vi "LV2015_PC_Build SD Card LED File from Page Cluser Array.vi"(7 "file path (dialog if empty)":path, 9 "pixel Count":u32=70, 11 "LED File Array":T1[](array[typedef])) -> ()   [LabVIEW 2016]
uses:
  TypeDefs/Cluster_Page Data.ctl
  <vilib>/Utility/file.llb/Write Delimited Spreadsheet (I64).vi
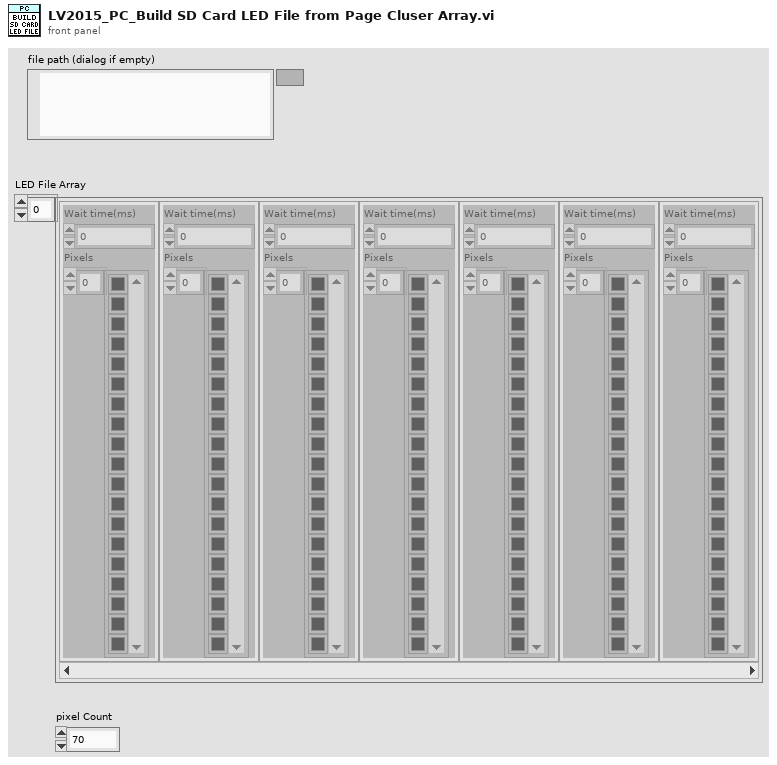
[diagram p1: front panel]
types:
  T1 = typedef "Cluster_Page Data.ctl" = cluster{"Wait time(ms)":u32, "Pixels":u32[]}
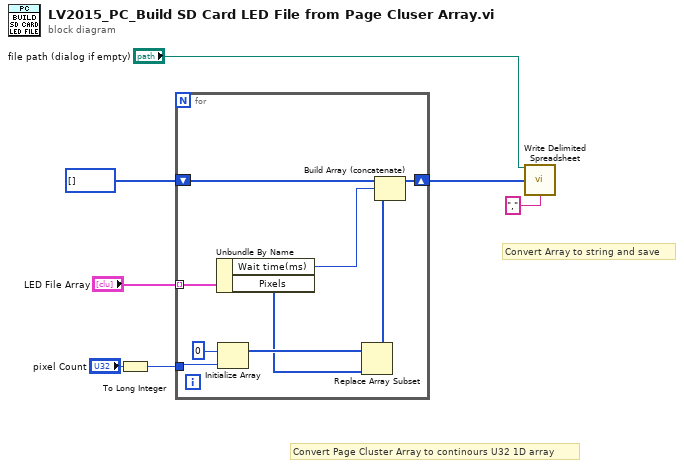
[diagram p0: block diagram]
diagram:
  # "Convert Array to string and save"
  # "Convert Page Cluster Array to continours U32 1D array"
  n1 = To Long Integer(number="pixel Count") -> (32bit integer=w4:i32)
  n2 = for {
    tunnel: "LED File Array" -> [w14] mode=indexing
    shift-right: [w10] -> w3
    shift-left: u32[] [] -> [w11]
    tunnel: w4 -> [w16]
    n3 = Unbundle By Name(w14) -> ("Wait time(ms)"=w9:u32, "Pixels"=w12:u32[])
    n4 = Initialize Array(u32 0 ("pixel Count 2"), w16) -> (w13:u32[])
    n5 = Replace Array Subset(array=w13, new element=w12) -> (w8:u32[])  [unwired: 1 in]
    n6 = Build Array (concatenate)(w11, w9, w8) -> (w10:u32[])
  }
  n7 = call-poly <vilib>:"Write Delimited Spreadsheet.vi"("file path (dialog if empty)"="file path (dialog if empty)", "1D data"=w3, "delimiter (\\t)"="," ("delimiter (\\t)")) -> ()  [unwired: 11 in, 2 out]
